vi "Initialize DAQmx Channels.vi"(8 "error in (no error)":errorcluster, 11 "Hardware Configuration In":T1={"Accel-ai0"=FALSE, "Maximum Input"=0.0, "Minimum Input"=0.0, "Sample Rate"=0.0, "Number of Samples"=0, "Accel-ai1"=FALSE, "DAQmx Task"="", "Low Pass Filter"={"Upper Cutoff"=350.0, "Lower Cutoff"=350.0, "Order"=350}} {"Low Pass Filter"."Order" min=0 max=10 step=1}) -> (0 "error out":errorcluster, 3 "Hardware Configuration Out":T1={"Accel-ai0"=FALSE, "Maximum Input"=0.0, "Minimum Input"=0.0, "Sample Rate"=0.0, "Number of Samples"=0, "Accel-ai1"=FALSE, "DAQmx Task"="", "Low Pass Filter"={"Upper Cutoff"=350.0, "Lower Cutoff"=350.0, "Order"=350}} {"Low Pass Filter"."Order" min=0 max=10 step=1})   [LabVIEW 2022 SP3, in "Acquisition.lvlib"]
doc: "Initialize the hardware references."
uses:
  Acquisition.lvlib
  FiniteMeasurement-DAQmx/controls/Hardware Configuration.ctl
  AcquisitionFilter.ctl
  FiniteMeasurement-DAQmx/controls/AccelerometerSettings.ctl
  <vilib>/DAQmx/create/channels.llb/DAQmx Create Channel (AI-Acceleration-Accelerometer).vi
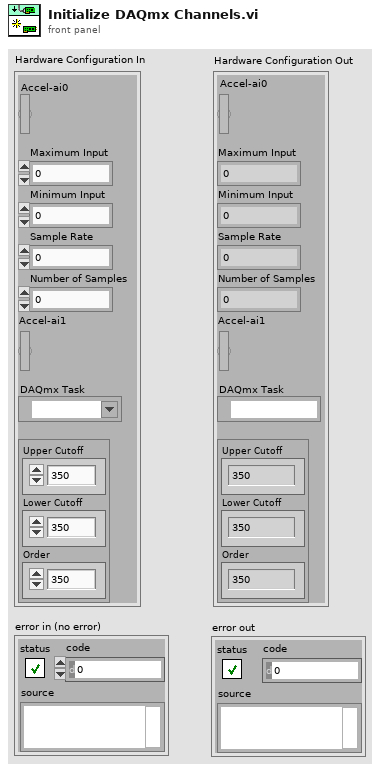
[diagram p1: front panel]
types:
  T1 = typedef "Acquisition.lvlib/Hardware Configuration.ctl" = cluster{"Accel-ai0":bool, "Maximum Input":dbl, "Minimum Input":dbl, "Sample Rate":dbl, "Number of Samples":i32, "Accel-ai1":bool, "DAQmx Task":refnum<k21>, "Low Pass Filter":T2}
  T2 = typedef "Acquisition.lvlib/AcquisitionFilter.ctl" = cluster{"Upper Cutoff":dbl, "Lower Cutoff":dbl, "Order":i32}
  T3 = typedef "AccelerometerSettings.ctl" = cluster{"current excitation source":i32, "current excitation value":dbl, "name to assign":string, "physical channels":tag, "sensitivity":dbl, "sensitivity units":i32, "units":i32}
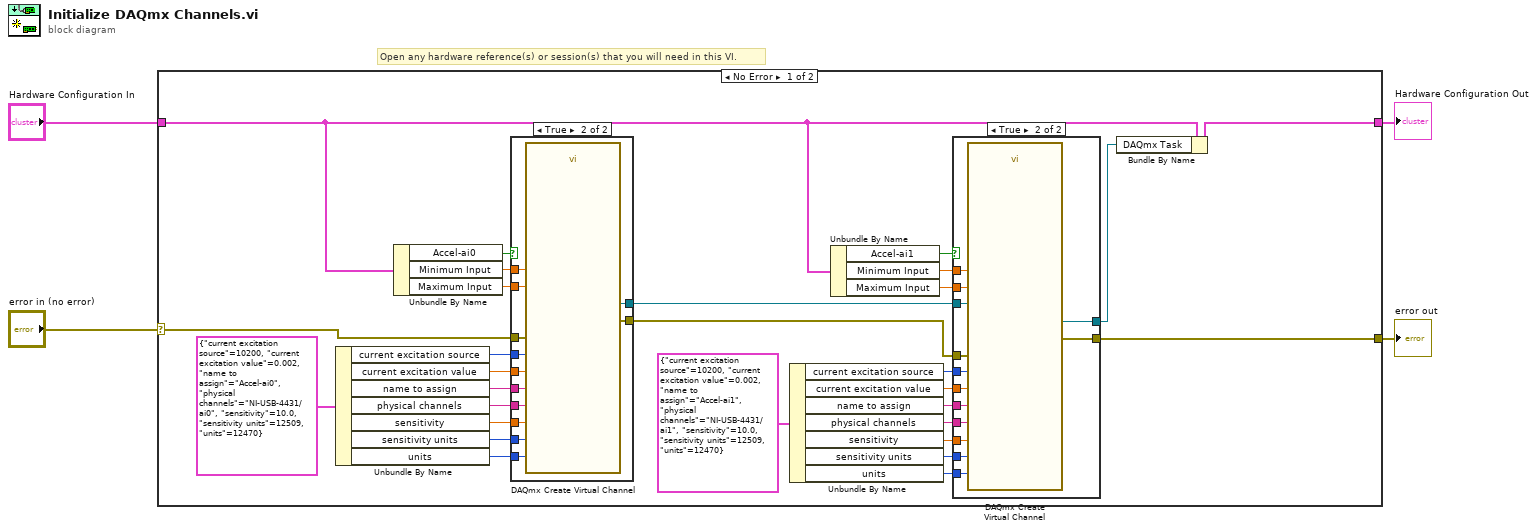
[diagram p0: block diagram]
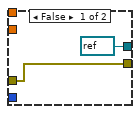
[diagram p3: hidden frame]
diagram:
  # "Open any hardware reference(s) or session(s) that you will need in this VI."
  n1 = case shown="No Error" "error in (no error)" {
    selector: "error in (no error)" -> [w9 w63]
    tunnel: [w8 w63] -> w3
    tunnel: "Hardware Configuration In" -> [w6 w64]
    tunnel: [w33 w64] -> w2
    frame No Error {
      n2 = Unbundle By Name(T3 {"current excitation source"=10200, "current excitation value"=0.002, "name to assign"="Accel-ai0", "physical channels"="NI-USB-4431/ai0", "sensitivity"=10.0, "sensitivity units"=12509, "units"=12470}) -> ("current excitation source"=w31:i32, "current excitation value"=w30:dbl, "name to assign"=w29:string, "physical channels"=w28:tag, "sensitivity"=w27:dbl, "sensitivity units"=w26:i32, "units"=w25:i32)
      n3 = Unbundle By Name(w6) -> ("Accel-ai0"=w10:bool, "Minimum Input"=w12:dbl, "Maximum Input"=w11:dbl)
      n4 = case shown="True" w10 {
        tunnel: w9 -> [w50 w62]
        tunnel: [w50 w61] -> w16
        tunnel: [refnum<k21> refnum ("task out") w60] -> w5
        tunnel: w31 -> [_ w59]
        tunnel: w30 -> [_ w58]
        tunnel: w29 -> [_ w57]
        tunnel: w28 -> [_ w56]
        tunnel: w27 -> [_ w55]
        tunnel: w26 -> [_ w54]
        tunnel: w25 -> [_ w53]
        tunnel: w12 -> [_ w52]
        tunnel: w11 -> [_ w51]
        frame False {
        }
        frame True {
          n5 = call-poly <vilib>:"DAQmx Create Virtual Channel.vi"("maximum value"=w51, "minimum value"=w52, "physical channels"=w56, "current excitation source"=w59, "name to assign"=w57, "current excitation value"=w58, "units"=w53, "error in"=w62, "sensitivity"=w55, "sensitivity units"=w54) -> ("task out"=w60:refnum<k21>, "error out"=w61:errorcluster)  [unwired: 4 in]
        }
      }
      n6 = Unbundle By Name(T3 {"current excitation source"=10200, "current excitation value"=0.002, "name to assign"="Accel-ai1", "physical channels"="NI-USB-4431/ai1", "sensitivity"=10.0, "sensitivity units"=12509, "units"=12470}) -> ("current excitation source"=w17:i32, "current excitation value"=w18:dbl, "name to assign"=w19:string, "physical channels"=w20:tag, "sensitivity"=w21:dbl, "sensitivity units"=w22:i32, "units"=w23:i32)
      n7 = Unbundle By Name(w6) -> ("Accel-ai1"=w13:bool, "Minimum Input"=w14:dbl, "Maximum Input"=w15:dbl)
      n8 = case shown="True" w13 {
        tunnel: [w35 w48] -> w7
        tunnel: w21 -> [_ w45]
        tunnel: w5 -> [w35 w47]
        tunnel: w23 -> [_ w40]
        tunnel: w22 -> [_ w46]
        tunnel: w20 -> [_ w44]
        tunnel: w19 -> [_ w43]
        tunnel: w18 -> [_ w42]
        tunnel: w17 -> [_ w41]
        tunnel: w16 -> [w34 w39]
        tunnel: [w34 w38] -> w8
        tunnel: w15 -> [_ w37]
        tunnel: w14 -> [_ w36]
        frame False {
        }
        frame True {
          n9 = call-poly <vilib>:"DAQmx Create Virtual Channel.vi"("task in"=w47, "maximum value"=w37, "minimum value"=w36, "physical channels"=w44, "current excitation source"=w41, "name to assign"=w43, "current excitation value"=w42, "units"=w40, "error in"=w39, "sensitivity"=w45, "sensitivity units"=w46) -> ("task out"=w48:refnum<k21>, "error out"=w38:errorcluster)  [unwired: 3 in]
        }
      }
      n10 = Bundle By Name(cluster=w6, "DAQmx Task"=w7) -> (w33:T1)
    }
    frame Error {
    }
  }
  "error out" <- w3
  "Hardware Configuration Out" <- w2
